vi "Handle Redirect.vi"(5 "Redirect URI":refnum<class "URI.lvclass">, 7 "Requested Scopes":string[](array[string]), 11 "Request in":refnum<class "Request.lvclass">) -> (0 "error out":errorcluster, 1 "Code":string, 2 "State Param":string)   [LabVIEW 2020, in "OAuth2.lvlib" / "OAuth2.lvclass"]
uses:
  OAuth2.lvclass
  OAuth2.lvclass/OAuth2.ctl
  HTTP Utils/Request/Request.lvclass
  <vilib>/IlluminatedG/lv-stream/URI/URI.lvclass
  OAuth2 Error.ctl
  OAuth2.lvlib
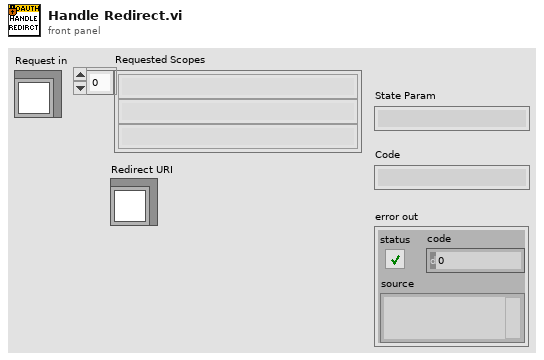
[diagram p1: front panel]
types:
  T1 = typedef "OAuth2.lvlib/OAuth2 Error.ctl" = enum16{"no_error", "admin_policy_enforced", "disallowed_useragent", "org_internal", "invalid_grant", "redirect_uri_mismatch"}
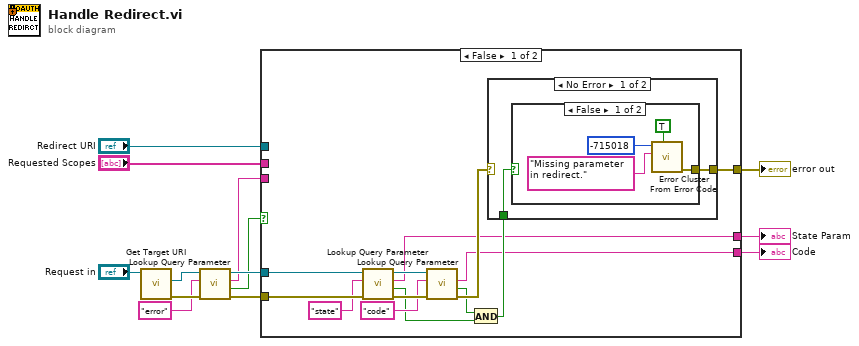
[diagram p0: block diagram]
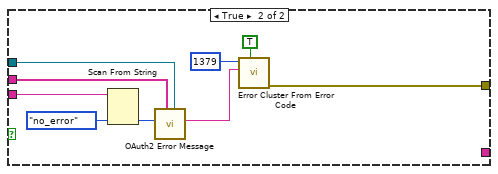
[diagram p4: hidden frame]
diagram:
  n1 = call "Get Target URI.vi"("Request in"="Request in") -> ("error out"=w10:errorcluster, "Target URI"=w11:refnum<class "URI.lvclass">)  [unwired: 8 in, 1 out]
  n2 = call <vilib>:"Lookup Query Parameter.vi"("error in (no error)"=w10, "Name"="error", "URI in"=w11) -> ("error out"=w13:errorcluster, "Found"=w6:bool, "Value"=w7:string, "URI out"=w9:refnum<class "URI.lvclass">)  [unwired: 5 in]
  n3 = case shown="False" w6 {
    tunnel: w13 -> [w25 _]
    tunnel: w9 -> [w18 _]
    tunnel: w7 -> [_ w41]
    tunnel: "Requested Scopes" -> [_ w39]
    tunnel: "Redirect URI" -> [_ w38]
    tunnel: [w17 w34] -> w3
    tunnel: [w15 _] -> w2
    tunnel: [w14 _] -> w1
    frame False {
      n4 = call <vilib>:"Lookup Query Parameter.vi"("error in (no error)"=w25, "Name"="state", "URI in"=w18) -> ("error out"=w22:errorcluster, "Found"=w20:bool, "Value"=w15:string, "URI out"=w23:refnum<class "URI.lvclass">)  [unwired: 5 in]
      n5 = call <vilib>:"Lookup Query Parameter.vi"("error in (no error)"=w22, "Name"="code", "URI in"=w23) -> ("error out"=w26:errorcluster, "Found"=w19:bool, "Value"=w14:string)  [unwired: 5 in, 1 out]
      n6 = And(x=w19, y=w20) -> (x .and. y?=w16:bool)
      n7 = case shown="No Error" w26 {
        selector: w26 -> [_ w33]
        tunnel: [w27 w33] -> w17
        tunnel: w16 -> [w28 _]
        frame No Error {
          n8 = case shown="False" w28 {
            tunnel: [w32 _] -> w27
            frame False {
              n9 = call <vilib>:"Error Cluster From Error Code.vi"("show call chain? (False)"=TRUE, "error message (\"\")"="Missing parameter in redirect.", "error code (0)"=-715018) -> ("error out"=w32:errorcluster)  [unwired: 6 in]
            }
            frame True {
            }
          }
        }
        frame Error {
        }
      }
    }
    frame True {
      n10 = Scan From String(input string=w41, default 1=OAuth2_Error."no_error" ("OAuth2 Error")) -> (output 1=w40:T1)  [unwired: 3 in, 3 out]
      n11 = call "OAuth2 Error Message.vi"("Redirect URI"=w38, "Requested Scopes"=w39, "OAuth2 Error"=w40) -> ("Error Message"=w36:string)  [unwired: 8 in]
      n12 = call <vilib>:"Error Cluster From Error Code.vi"("show call chain? (False)"=TRUE, "error message (\"\")"=w36, "error code (0)"=1379) -> ("error out"=w34:errorcluster)  [unwired: 6 in]
    }
  }
  "error out" <- w3
  "Code" <- w1
  "State Param" <- w2
